vi "esp save positions to db.vi"(8 "error in (no error)":errorcluster, 11 "ESP301 in":refnum<class "ESP301.lvclass">) -> (0 "error out":errorcluster, 3 "ESP301 out":refnum<class "ESP301.lvclass">)   [LabVIEW 2020, in "ESP301.lvclass"]
uses:
  ESP301.lvclass
  ESP301.lvclass/ESP301.ctl
panel:
  out "x-y":u32
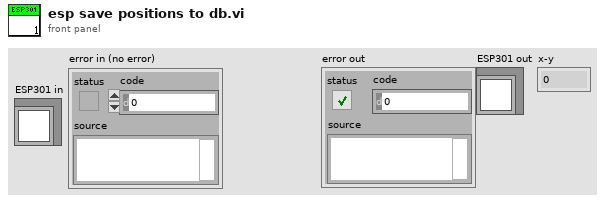
[diagram p1: front panel]
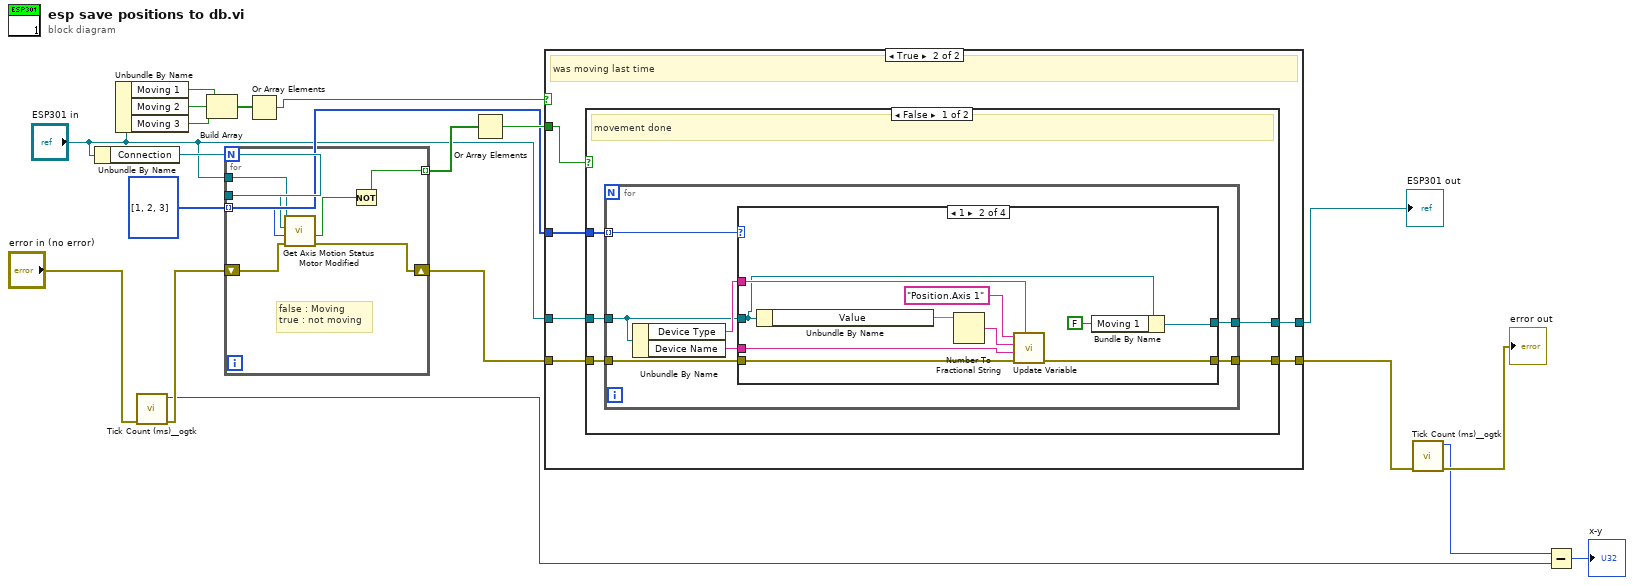
[diagram p0: block diagram]
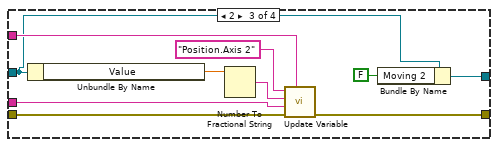
[diagram p4: hidden frame]
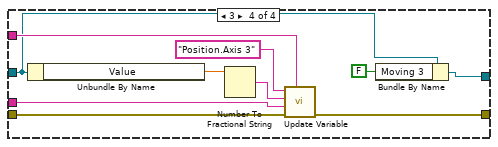
[diagram p5: hidden frame]
diagram:
  w16 = i32[] [1, 2, 3]
  n1 = Unbundle By Name("ESP301 in") -> ("Connection"=w17:refnum<visa-resource-name>)
  n2 = Unbundle By Name("ESP301 in") -> ("Moving 1"=w13:bool, "Moving 2"=w12:bool, "Moving 3"=w11:bool)
  n3 = call <userlib>:"Tick Count (ms)__ogtk.vi"("error in (no error)"="error in (no error)") -> ("error out"=w4:errorcluster, "millisecond timer value"=w2:u32)  [unwired: 9 in]
  n4 = Build Array(w13, w12, w11) -> (w10:bool[])
  n5 = for {
    tunnel: "ESP301 in" -> [w24]
    tunnel: w17 -> [w23]
    shift-right: [w25] -> w18
    shift-left: w4 -> [w26]
    tunnel: w16 -> [w22] mode=indexing
    tunnel: [w21] -> w15 mode=indexing
    # "false : Moving\ntrue : not moving"
    n6 = call-dynamic "Get Axis Motion Status Motor Modified.vi"("error in (no error)"=w26, "Axis (1)"=w22, "VISA resource name"=w23, "ESP301 in"=w24) -> ("error out"=w25:errorcluster, "Motion Done"=w20:bool)  [unwired: 4 in, 2 out]
    n7 = Not(x=w20) -> (.not. x?=w21:bool)
  }
  n8 = Or Array Elements(Boolean array=w10) -> (logical OR=w9:bool)
  n9 = Or Array Elements(Boolean array=w15) -> (logical OR=w19:bool)
  n10 = case shown="True" w9 {
    tunnel: w19 -> [_ w34]
    tunnel: "ESP301 in" -> [w27 w33]
    tunnel: w18 -> [w28 w32]
    tunnel: [w28 w31] -> w6
    tunnel: w16 -> [_ w30]
    tunnel: [w27 w29] -> w8
    frame False {
      # "was not moving last time"
    }
    frame True {
      # "was moving last time"
      n11 = case shown="False" w34 {
        tunnel: w33 -> [w39 w79]
        tunnel: w32 -> [w38 w80]
        tunnel: [w37 w80] -> w31
        tunnel: w30 -> [w36 _]
        tunnel: [w35 w79] -> w29
        frame False {
          # "movement done"
          n12 = for {
            tunnel: w36 -> [w46] mode=indexing
            tunnel: w39 -> [w41]
            tunnel: w38 -> [w43]
            tunnel: [w42] -> w37
            tunnel: [w40] -> w35
            n13 = Unbundle By Name(w41) -> ("Device Type"=w45:string, "Device Name"=w44:string)
            n14 = case shown="1" w46 {
              tunnel: w41 -> [w47 w50 w60 w70]
              tunnel: [w48 w57 w67 w77] -> w42
              tunnel: w45 -> [_ w54 w64 w74]
              tunnel: w44 -> [_ w53 w63 w73]
              tunnel: w43 -> [w48 w52 w62 w72]
              tunnel: [w47 w49 w59 w69] -> w40
              frame 0, Default {
              }
              frame 1 {
                n15 = Unbundle By Name(w50) -> ("Value"=w56:dbl)
                n16 = Number To Fractional String(number=w56) -> (F-format string=w55:string)  [unwired: 3 in]
                n17 = call "Update Variable.vi"("Device Type"=w54, "error in (no error)"=w52, "device name"=w53, "Variable Value"=w55, "Variable Name"="Position.Axis 1" ("Variable Value")) -> ("error out"=w57:errorcluster)  [unwired: 6 in]
                n18 = Bundle By Name(cluster=w50, "Moving 1"=FALSE) -> (w49:refnum<class "ESP301.lvclass">)
              }
              frame 2 {
                n19 = Unbundle By Name(w60) -> ("Value"=w66:dbl)
                n20 = Number To Fractional String(number=w66) -> (F-format string=w65:string)  [unwired: 3 in]
                n21 = call "Update Variable.vi"("Device Type"=w64, "error in (no error)"=w62, "device name"=w63, "Variable Value"=w65, "Variable Name"="Position.Axis 2" ("Variable Value")) -> ("error out"=w67:errorcluster)  [unwired: 6 in]
                n22 = Bundle By Name(cluster=w60, "Moving 2"=FALSE ("Moving 1")) -> (w59:refnum<class "ESP301.lvclass">)
              }
              frame 3 {
                n23 = Unbundle By Name(w70) -> ("Value"=w76:dbl)
                n24 = Number To Fractional String(number=w76) -> (F-format string=w75:string)  [unwired: 3 in]
                n25 = call "Update Variable.vi"("Device Type"=w74, "error in (no error)"=w72, "device name"=w73, "Variable Value"=w75, "Variable Name"="Position.Axis 3" ("Variable Value")) -> ("error out"=w77:errorcluster)  [unwired: 6 in]
                n26 = Bundle By Name(cluster=w70, "Moving 3"=FALSE ("Moving 1")) -> (w69:refnum<class "ESP301.lvclass">)
              }
            }
          }
        }
        frame True {
          # "still moving"
        }
      }
    }
  }
  "ESP301 out" <- w8
  n27 = call <userlib>:"Tick Count (ms)__ogtk.vi"("error in (no error)"=w6) -> ("error out"=→"error out":errorcluster, "millisecond timer value"=w3:u32)  [unwired: 9 in]
  n28 = Subtract(x=w3, y=w2) -> (x-y=→"x-y":u32)
